vi "CRYTS Tree Fresh.vi"(0 "SequenceTree":refnum<vi>, 1 "Edit Index":i32, 5 "sOption":string, 7 "Source Index":i32, 9 "SourceCount":i32, 11 "Target Index":i32, 12 "Is Refresh?":bool=TRUE) -> (4 "SequenceTree out":refnum<vi>)   [LabVIEW 2013]
uses:
  <vilib>/Utility/miscctls.llb/LVNodeAndColumnTypeDef.ctl
  CRYProject Editor Global.vi
panel:
  in  "Temp No":i32
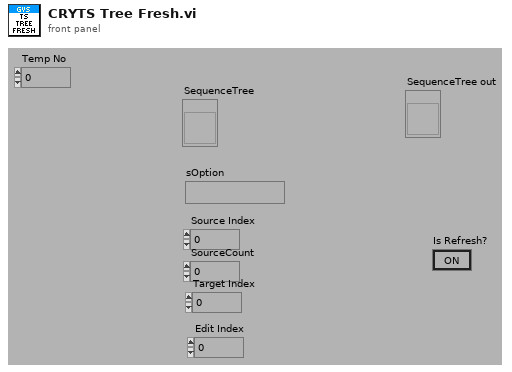
[diagram p1: front panel]
types:
  T1 = typedef "CRYTS.ctl" = cluster{"No.TS":u16, "TS File Path":path, "TS Name":string, "EditStepName":string, "Steps":T2[], "New State":bool, "Change State":bool, "Flattened CurveLib Data":string, "Document Data":string, "EditStepNo":u16, "Operator Start File":string, "Sequence Type":string, "Sequence Language":string}
  T2 = typedef "CRYStep.ctl" = cluster{"No.VI":i32, "Category":string, "StepName":string, "Seq setup flattened":string, "Comment":string, "Steps config.":bool[], "Jump config":i32[], "Start":dbl, "Increment":dbl, "Name":string, "Unit":string, "Y data":u16, "Y prefix":string, "Y dB ref":dbl, "Y unit":string, "Repeat State Array":cluster{"Start":dbl, "Increment":dbl, "Count":i32, "Num":i32}[]}
  T3 = cluster{"Left Cell String":string, "Child Text":string[], "Child Tag":string, "Item Indent":i32, "Child Only?":bool, "Glyph Index":i32}[]
  T4 = typedef "LVNodeAndColumnTypeDef.ctl" = cluster{"Node":string, "Column":i32}
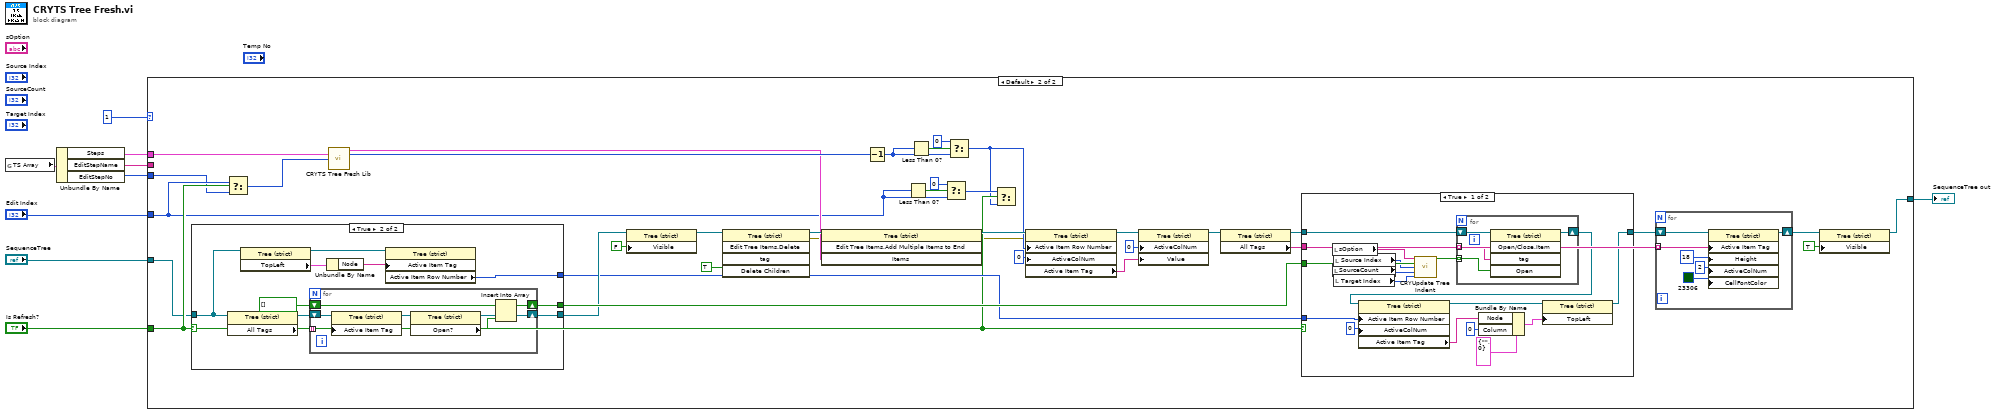
[diagram p0: block diagram]
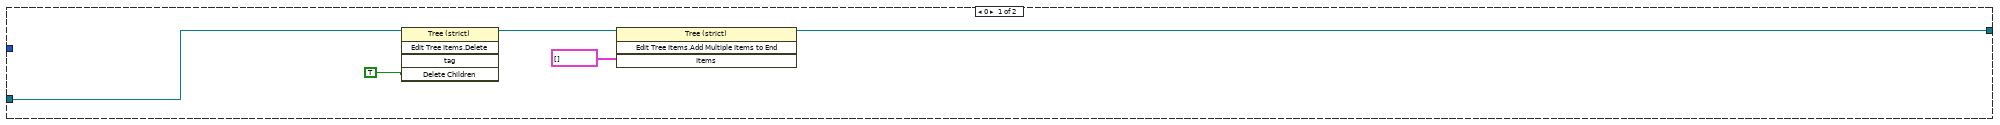
[diagram p2: hidden frame]
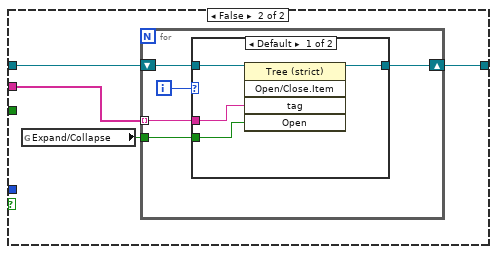
[diagram p3: hidden frame]
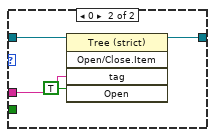
[diagram p4: hidden frame]
diagram:
  n1 = global read "CRYProject Editor Global.vi" "TS Array"() -> (w5:T1)
  n2 = Unbundle By Name(w5) -> ("Steps"=w9:T2[], "EditStepName"=w7:string, "EditStepNo"=w2:u16)
  n3 = case shown="Default" 1 ("size(s)") {
    tunnel: "SequenceTree" -> [w11 w15]
    tunnel: w9 -> [_ w28]
    tunnel: w7 -> [_ _]
    tunnel: [w10 w38] -> w6
    tunnel: "Is Refresh?" -> [_ w22]
    tunnel: w2 -> [_ w20]
    tunnel: "Edit Index" -> [_ w21]
    frame 0 {
      n4 = invoke on="Invoke Node" class="Tree (strict)" method="Edit Tree Items.Delete"(reference=w11, "Delete Children"=TRUE ("Delete Children?")) -> (reference out=w13:refnum<vi>)  [unwired: 3 in, 4 out]
      n5 = invoke class="Tree (strict)" method="Edit Tree Items.Add Multiple Items to End"(reference=w13, "Items"=T3 []) -> (reference out=w10:refnum<vi>)  [unwired: 2 in, 3 out]
    }
    frame Default {
      n6 = case shown="True" w22 {
        tunnel: [_ w105] -> w46
        tunnel: w15 -> [w95 w100]
        tunnel: [w95 w102] -> w44
        tunnel: [_ w99] -> w31
        frame False {
        }
        frame True {
          n7 = property class="Tree (strict)"(reference=w100) -> (reference out=w104:refnum<vi>, "All Tags"=w101:string[])  [unwired: 1 in, 1 out]
          n8 = property class="Tree (strict)"(reference=w100) -> (reference out=w97:refnum<vi>, "TopLeft"=w98:T4)  [unwired: 1 in, 1 out]
          n9 = for {
            tunnel: w101 -> [w107] mode=indexing
            shift-right: [w108] -> w105
            shift-left: bool[] [] ("Array") -> [w109]
            shift-right: [w106] -> w102
            shift-left: w104 -> [w111]
            n10 = property class="Tree (strict)"(reference=w111, "Active Item Tag"=w107) -> (reference out=w112:refnum<vi>)  [unwired: 1 in, 1 out]
            n11 = property class="Tree (strict)"(reference=w112) -> (reference out=w106:refnum<vi>, "Open?"=w110:bool)  [unwired: 1 in, 1 out]
            n12 = Insert Into Array(array=w109, new element=w110) -> (w108:bool[])  [unwired: 1 in]
          }
          n13 = Unbundle By Name(w98) -> ("Node"=w96:string)
          n14 = property on="Property Node" class="Tree (strict)"(reference=w97, "Active Item Tag"=w96) -> ("Active Item Row Number"=w99:i32)  [unwired: 1 in, 2 out]
        }
      }
      n15 = Select(t=w21, s=w22, f=w20) -> (s? t:f=w19:i32)
      n16 = call "CRYTS Tree Fresh Lib.vi"("Steps"=w28, "EditStepNo"=w19) -> ("Tree Items"=w26:T3, "Edit Step Index"=w27:i32)  [unwired: 12 in]
      n17 = property class="Tree (strict)"(reference=w44, "Visible"=FALSE) -> (reference out=w48:refnum<vi>)  [unwired: 1 in, 1 out]
      n18 = invoke on="Invoke Node" class="Tree (strict)" method="Edit Tree Items.Delete"(reference=w48, "Delete Children"=TRUE ("Delete Children?")) -> (reference out=w49:refnum<vi>, error out=w16:errorcluster)  [unwired: 3 in, 3 out]
      n19 = invoke class="Tree (strict)" method="Edit Tree Items.Add Multiple Items to End"(reference=w49, error in=w16, "Items"=w26) -> (reference out=w40:refnum<vi>, error out=w17:errorcluster)  [unwired: 1 in, 2 out]
      n20 = Decrement(x=w27) -> (x-1=w42:i32)
      n21 = Less Than 0?(x=w21) -> (x < 0?=w35:bool)
      n22 = Less Than 0?(x=w42) -> (x < 0?=w43:bool)
      n23 = Select(t=0, s=w35, f=w21) -> (s? t:f=w32:i32)
      n24 = Select(t=0, s=w43, f=w42) -> (s? t:f=w18:i32)
      n25 = Select(t=w32, s=w22, f=w18) -> ()  [unwired: 1 out]
      n26 = property on="Property Node" class="Tree (strict)"(reference=w40, error in=w17, "Active Item Row Number"=w18, "ActiveColNum"=0 ("Active Cell:Active Column Number")) -> (reference out=w39:refnum<vi>, "Active Item Tag"=w37:string)  [unwired: 1 out]
      n27 = property class="Tree (strict)"(reference=w39, "ActiveColNum"=0 ("Active Cell:Active Column Number"), "Value"=w37) -> (reference out=w29:refnum<vi>)  [unwired: 1 in, 1 out]
      n28 = property class="Tree (strict)"(reference=w29) -> (reference out=w30:refnum<vi>, "All Tags"=w24:string[])  [unwired: 1 in, 1 out]
      n29 = case shown="True" w22 {
        tunnel: [w66 w81] -> w25
        tunnel: w46 -> [w72 _]
        tunnel: w30 -> [w68 w80]
        tunnel: w24 -> [w70 w79]
        tunnel: w31 -> [w65 _]
        frame True {
          n30 = local read "sOption"() -> (w73:string)
          n31 = local read "SourceCount"() -> (w69:i32)
          n32 = local read "Source Index"() -> (w64:i32)
          n33 = local read "Target Index"() -> (w63:i32)
          n34 = call "CRYUpdate Tree Indent.vi"("sOption"=w73, "Open States In"=w72, "Source Index"=w64, "SourceCount"=w69, "Target Index"=w63) -> ("Open States Out"=w71:bool[])  [unwired: 10 in]
          n35 = for {
            tunnel: w71 -> [w77] mode=indexing
            tunnel: w70 -> [w74] mode=indexing
            shift-right: [w76] -> w67
            shift-left: w68 -> [w75]
            n36 = invoke class="Tree (strict)" method="Open/Close.Item"(reference=w75, "tag"=w74, "Open"=w77) -> (reference out=w76:refnum<vi>)  [unwired: 2 in, 4 out]
          }
          n37 = property on="Property Node" class="Tree (strict)"(reference=w67, "Active Item Row Number"=w65, "ActiveColNum"=0 ("Active Cell:Active Column Number")) -> (reference out=w59:refnum<vi>, "Active Item Tag"=w58:string)  [unwired: 1 in, 1 out]
          n38 = Bundle By Name(cluster=T4 {"Node"="", "Column"=0} ("Top Left Visible Cell"), "Node"=w58, "Column"=0) -> (w60:T4)
          n39 = property class="Tree (strict)"(reference=w59, "TopLeft"=w60) -> (reference out=w66:refnum<vi>)  [unwired: 1 in, 1 out]
        }
        frame False {
          n40 = global read "CRYProject Editor Global.vi" "Expand/Collapse"() -> (w78:bool)
          n41 = for {
            tunnel: w79 -> [w84] mode=indexing
            shift-right: [w86] -> w81
            shift-left: w80 -> [w85]
            tunnel: w78 -> [w82]
            i -> [w83]
            n42 = case shown="Default" w83 {
              tunnel: [w89 w94] -> w86
              tunnel: w85 -> [w90 w93]
              tunnel: w84 -> [w88 w92]
              tunnel: w82 -> [w87 _]
              frame Default {
                n43 = invoke class="Tree (strict)" method="Open/Close.Item"(reference=w90, "tag"=w88, "Open"=w87) -> (reference out=w89:refnum<vi>)  [unwired: 2 in, 4 out]
              }
              frame 0 {
                n44 = invoke class="Tree (strict)" method="Open/Close.Item"(reference=w93, "tag"=w92, "Open"=TRUE ("Open?")) -> (reference out=w94:refnum<vi>)  [unwired: 2 in, 4 out]
              }
            }
          }
        }
      }
      n45 = for {
        tunnel: w24 -> [w53] mode=indexing
        shift-right: [w55] -> w23
        shift-left: w25 -> [w54]
        n46 = property class="Tree (strict)"(reference=w54, "Active Item Tag"=w53, "Height"=18 ("Active Cell:Cell Size:Height"), "ActiveColNum"=2 ("Active Cell:Active Column Number"), "CellFontColor"=u32 23306) -> (reference out=w55:refnum<vi>)  [unwired: 1 in, 1 out]
      }
      n47 = property class="Tree (strict)"(reference=w23, "Visible"=TRUE) -> (reference out=w38:refnum<vi>)  [unwired: 1 in, 1 out]
    }
  }
  "SequenceTree out" <- w6
